vi "A_SIG.vi"(3 "Cluster":T1, 5 "error in (no error)":errorcluster, 8 "Input":dbl) -> (16 "A_SIG_out":dbl, 19 "error out":errorcluster)   [LabVIEW 2022 SP3]
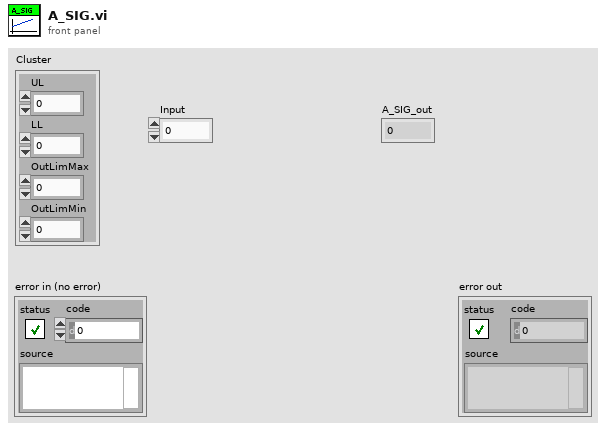
[diagram p1: front panel]
types:
  T1 = cluster{"UL":dbl, "LL":dbl, "OutLimMax":dbl, "OutLimMin":dbl}
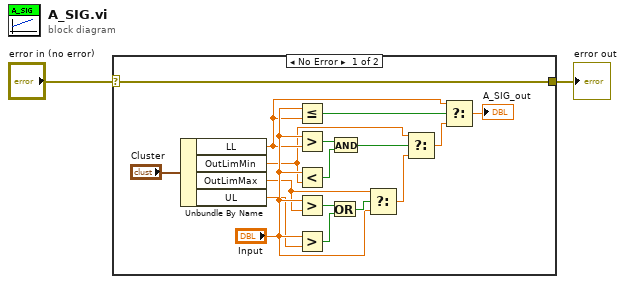
[diagram p0: block diagram]
diagram:
  n1 = case shown="No Error" "error in (no error)" {
    selector: "error in (no error)" -> [w19 w20]
    tunnel: [w19 w20] -> w1
    frame No Error {
      n2 = Unbundle By Name("Cluster") -> ("LL"=w6:dbl, "OutLimMin"=w5:dbl, "OutLimMax"=w4:dbl, "UL"=w3:dbl)
      n3 = Less Or Equal?(x="Input", y=w6) -> (x <= y?=w18:bool)
      n4 = Greater?(x="Input", y=w6) -> (0:w17:bool)
      n5 = Less?(x="Input", y=w5) -> (x < y?=w16:bool)
      n6 = Greater?(x="Input", y=w4) -> (0:w14:bool)
      n7 = Greater?(x="Input", y=w3) -> (0:w13:bool)
      n8 = Or(x=w14, y=w13) -> (x .or. y?=w12:bool)
      n9 = And(x=w17, y=w16) -> (x .and. y?=w15:bool)
      n10 = Select(t=w4, s=w12, f="Input") -> (s? t:f=w10:dbl)
      n11 = Select(t=w5, s=w15, f=w10) -> (s? t:f=w9:dbl)
      n12 = Select(t=w6, s=w18, f=w9) -> (s? t:f=→"A_SIG_out":dbl)
    }
    frame Error {
    }
  }
  "error out" <- w1
